vi "Get Crafting Stations.vi"(8 "error in (no error)":errorcluster, 11 "Simple Case in":refnum<class "Simple Case.lvclass">) -> (0 "error out":errorcluster, 2 "Stations":T1[](array[typedef]), 3 "Simple Case out":refnum<class "Simple Case.lvclass">)   [LabVIEW 2020, in "Simple Case.lvclass"]
uses:
  Simple Case.lvclass
  Item/Craft Station.ctl
  Workstation/Workstation.lvclass
  Tinker Table/Tinker Table.lvclass
  C:/dev/IlluminatedG/lv-oopanel-gc-calc/Workstation/Workstation.lvclass
  Item/Item.lvclass
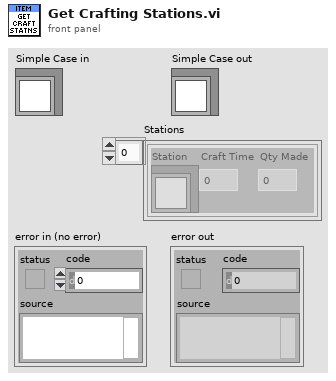
[diagram p1: front panel]
types:
  T1 = typedef "Item.lvclass/Craft Station.ctl" = cluster{"Station":refnum<class "Workstation.lvclass">, "Craft Time":dbl, "Qty Made":dbl}
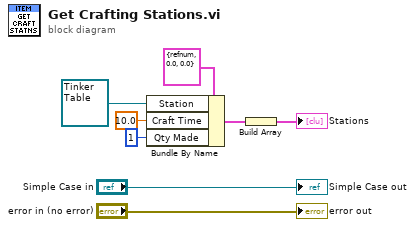
[diagram p0: block diagram]
diagram:
  n1 = Bundle By Name(cluster=T1 {"Station"=refnum, "Craft Time"=0.0, "Qty Made"=0.0} ("Craft Station"), "Station"=refnum<class "Tinker Table.lvclass"> refnum ("Tinker Table.lvclass"), "Craft Time"=10.0, "Qty Made"=1) -> (w5:T1)
  n2 = Build Array(w5) -> (→"Stations":T1[])
  "error out" <- "error in (no error)"
  "Simple Case out" <- "Simple Case in"
